vi "parse_Pose2D.vi"(4 "error in":errorcluster, 7 "msg in":string) -> (0 "error out":errorcluster, 2 "Pose 2D":cluster{"x":dbl, "y":dbl, "theta":dbl}, 3 "msg out":string)   [LabVIEW 2012]
doc: "Parses a message into a pose 2D"
uses:
  <userlib>/ROS for LabVIEW Software/ROS/MessageParsing/std_msgs/subs/parse_float64_scalar.vi
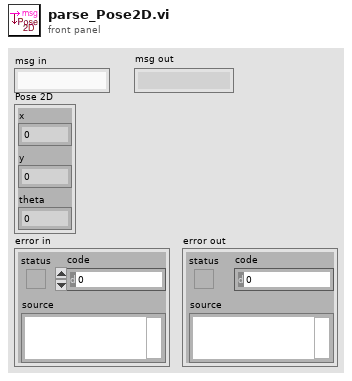
[diagram p1: front panel]
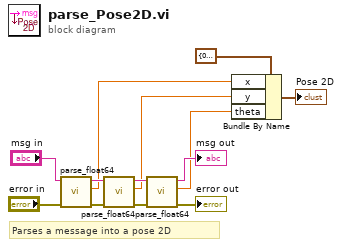
[diagram p0: block diagram]
diagram:
  # "Parses a message into a pose 2D"
  n1 = call-poly <userlib>:"parse_float64.vi"("error in"="error in", "msg in"="msg in") -> ("error out"=w10:errorcluster, "number"=w3:dbl, "msg out"=w11:string)  [unwired: 3 in]
  n2 = call-poly <userlib>:"parse_float64.vi"("error in"=w10, "msg in"=w11) -> ("error out"=w8:errorcluster, "number"=w2:dbl, "msg out"=w9:string)  [unwired: 3 in]
  n3 = call-poly <userlib>:"parse_float64.vi"("error in"=w8, "msg in"=w9) -> ("error out"=→"error out":errorcluster, "number"=w1:dbl, "msg out"=→"msg out":string)  [unwired: 3 in]
  n4 = Bundle By Name(cluster=cluster{"x":dbl, "y":dbl, "theta":dbl} {"x"=0.0, "y"=0.0, "theta"=0.0} ("input cluster"), "x"=w3, "y"=w2, "theta"=w1) -> (→"Pose 2D":cluster{"x":dbl, "y":dbl, "theta":dbl})
